vi "FXP_AFMss_LinearDistEst_singleAxis.vi"() -> ()   [LabVIEW 2017]
uses:
  typeDefs/FXPControlParams_distEst.ctl
  fpga_fp_interface_lib/fpga_interface_types/boolean_indicators.ctl
  <vilib>/Platform/TimedLoop/XDataNode/timing_clust.ctl
  <vilib>/Platform/TimedLoop/XDataNode/nitl_modes.ctl
  <vilib>/Platform/TimedLoop/XDataNode/wakeup.ctl
  <vilib>/rvi/Emulation/niFpgaSctlEmulationGetInTimedLoop.vi
  <vilib>/rvi/Emulation/niFpgaProcessEmulError.vi
  <vilib>/rvi/Emulation/niFpgaGetClockAttributes.vi
  <vilib>/rvi/Emulation/niFpgaEmulationReportErrorSimple.vi
  <vilib>/rvi/eio/common/nirviEmuTemplateMethod_errors.vi
  <vilib>/rvi/Emulation/niFpgaCriticalErrorInLSC.vi
  <vilib>/rvi/Memory/Memory_Emulation/nirvimemoryFastEmulation.vi
  <vilib>/rvi/Memory/Memory_Emulation/nirvimemoryEmulation.vi
  <vilib>/rvi/Emulation/niFpgaEmulationIsFPGAContextNoSignature.vi
  <vilib>/rvi/DataTransferAndStorage/Container/Common/niFpgaContainerGetUniqueNameForEmu.vi
  <vilib>/rvi/errors/nirviReportUnexpectedCaseInternalError (U32).vi
  <vilib>/rvi/interface/RandomDataEmulation/niFpgaRandomDataHandleErrors.vi
  <vilib>/eio/EIONode/EIONode.xnode
  <vilib>/Platform/TimedLoop/XDataNode/XDataNode.xnode
  <vilib>/rvi/DataTransferAndStorage/Container/XNode/niFpgaContainer.xnode
  <vilib>/rvi/interface/RandomDataEmulation/nirviRandomDataFpgaReadWriteTemplate.vi
  <vilib>/rvi/FXPMathLib/FxpSub/XNode/nifxpmath_Sub.xnode
  <vilib>/Platform/TimedLoop/XDataNode/XDNodeRunTimeDep.lvlib
  <vilib>/rvi/FXPMathLib/sim/FxpSim.dll
panel:
  out "u_k (saturated)":fxp<+/-,32,5>
  out "del u(k)":fxp<+/-,64,15>
  in  "N_sat":u8
  in  "N_hyst":u8
  in  "Num":sgl[](array[numeric])=[-0.00254, 0.000408, 0.00295, 0.0, 0.0, 0.0, 0.0, 0.0, 0.0]
  in  "Den":sgl[](array[numeric])=[0.982758, -1.98194, 1.0, 0.0, 0.0, 0.0, 0.0, 0.0, 0.0]
  in  "TF Order":i32=2
  out "SS FIFO TimeOut?":bool
  out "u_k":fxp<+/-,32,5>
  out "boolean indicators":T1
  in  "ControlParamsMpc":T2={"umax"=3.0, "Ns_obs/cntrl"=0, "ref_f_VEC"=[0.0, 0.0], "du_max"=0.0, "Nbar"=0.0}
  out "x(0)":fxp<+/-,16,5>
  out "Stopped":bool
  in  "Settle Ticks":i16=1000
  in  "iters":i32=1
  in  "ymax":fxp<+/-,32,16>=4.0
  in  "TsTicks":i16
  out "Loop Ticks (benchmark)":i16
  out "NS_O/C":u8=2
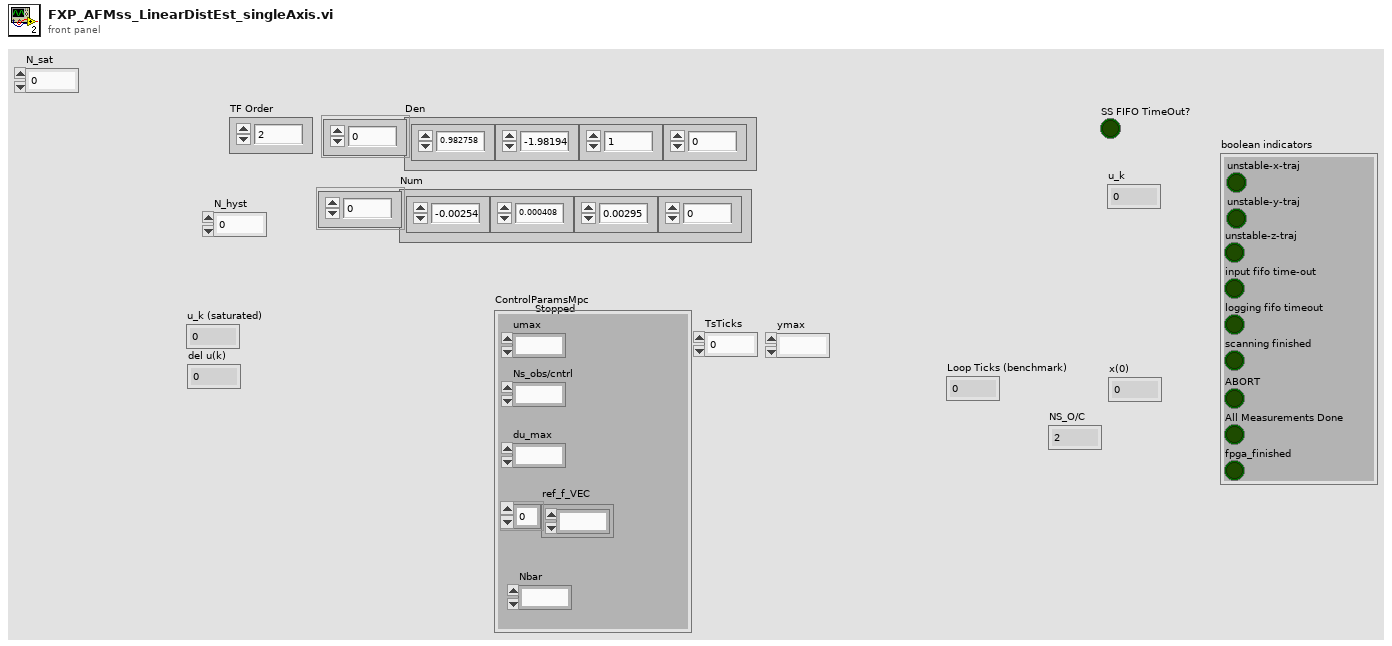
[diagram p1: front panel]
types:
  T1 = typedef "boolean_indicators.ctl" = cluster{"unstable-z-traj":bool, "input fifo time-out":bool, "logging fifo timeout":bool, "scanning finished":bool, "unstable-x-traj":bool, "unstable-y-traj":bool, "ABORT":bool, "All Measurements Done":bool, "fpga_finished":bool}
  T2 = typedef "FXPControlParams_distEst.ctl" = cluster{"umax":fxp<+/-,18,5>, "Ns_obs/cntrl":u8, "ref_f_VEC":fxp<+/-,32,5>[], "du_max":fxp<+/-,18,5>, "Nbar":fxp<+/-,32,5>}
  T3 = typedef "XDNodeRunTimeDep.lvlib/timing_clust.ctl" = cluster{"Expected End [f-1]":u64, "Actual End [f-1]":u64, "Finished Late? [f-1]":bool, "Expected End [i-1]":u64, "Actual End [i-1]":u64, "Finished Late? [i-1]":bool, "Expected Start [i]":u64, "Actual Start [i]":u64, "Expected Start [f]":u64, "Actual Start [f]":u64, "Source Name":string, "Structure Name":string, "Period":i64, "Deadline":i64, "Offset":i64, "Start":i64, "Priority":i32, "Timeout":i32, "Mode":T4, "Wakeup Reason":T5, "Error":errorcluster, "Source Type":string, "Secondary Source Type":string, "Global End Time":u64, "Global Start Time":u64, "Frame Duration":u64, "Iteration Duration":u64, "Assigned CPU":i32, "I/O Scan Engine Mode":u32}
  T4 = typedef "XDNodeRunTimeDep.lvlib/nitl_modes.ctl" = enum32{"No Change", "Process missed periods, maintain original phase", "Discard missed periods, maintain original phase", "Process missed periods, ignore original phase", "Discard missed periods, ignore original phase"}
  T5 = typedef "XDNodeRunTimeDep.lvlib/wakeup.ctl" = enum32{"Normal", "Aborted", "Asynchronous wakeup", "Timing source error", "Timed loop error", "Timeout"}
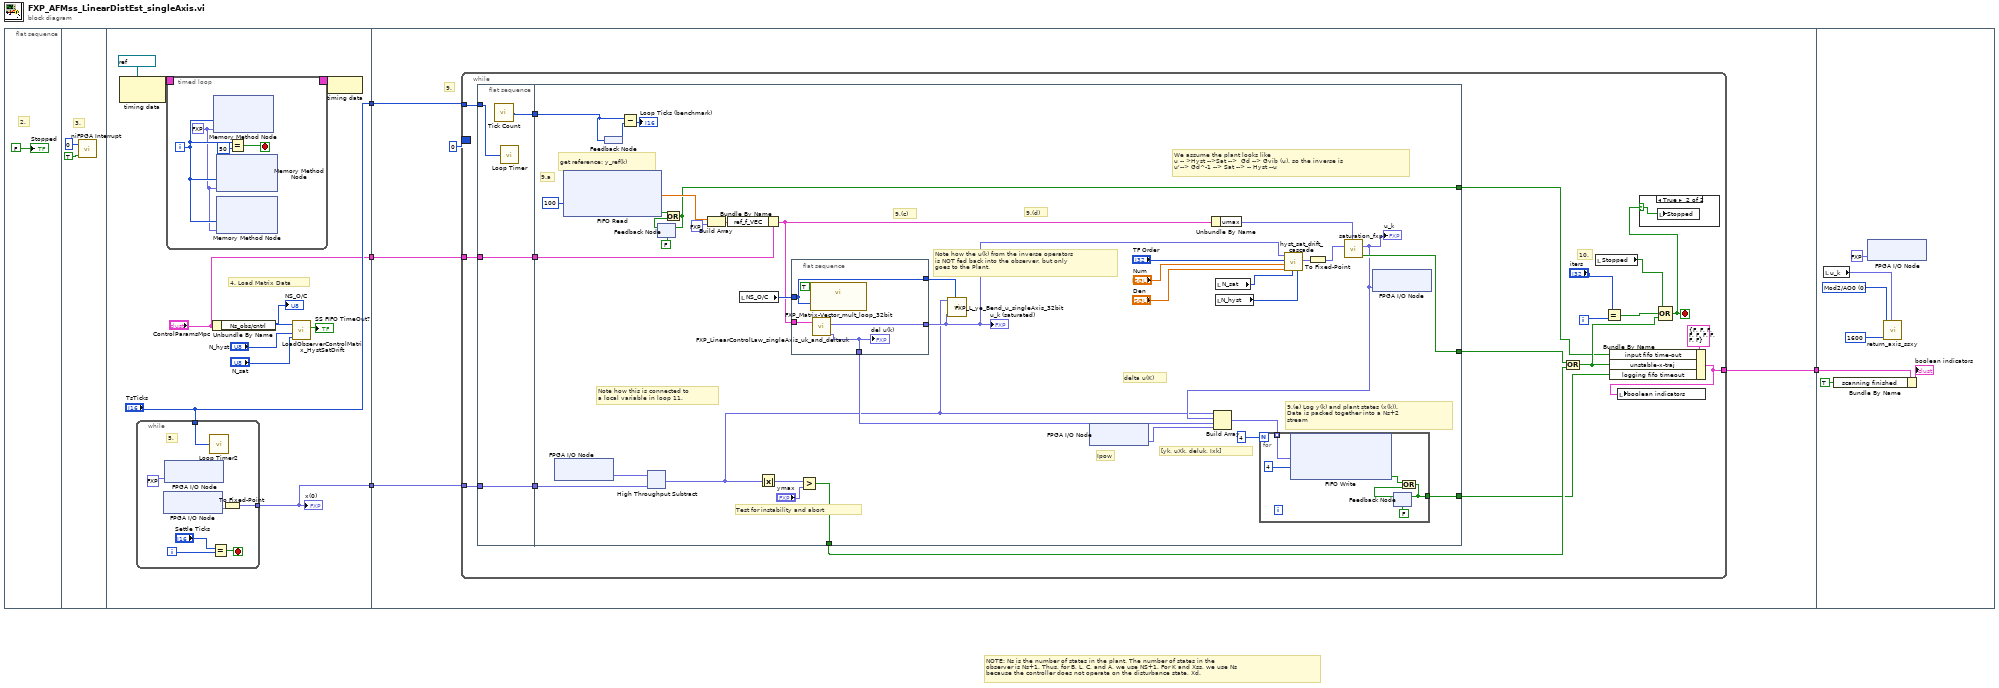
[diagram p0: block diagram]
diagram:
  # "NOTE: Ns is the number of states in the plant. The number of states in the \nobserver is Ns+1. Thus, for B, L, C, and A, we use NS+1. For K and Xss, we use Ns\nbecause the controller does not operate on the disturbance state, Xd."
  n1 = flat-sequence {
    tunnel: ["TsTicks"] -> w4
    tunnel: [w17] -> w3
    tunnel: ["ControlParamsMpc"] -> w2
    tunnel: w4 -> [w39]
    tunnel: w3 -> [w38]
    tunnel: w2 -> [w37]
    tunnel: [w36] -> w1
    tunnel: w1 -> [w116]
    frame #0 {
      # "2."
      "Stopped" <- FALSE ("Stopped")
    }
    frame #1 {
      # "3."
      n2 = call <vilib>:"niFPGA Interrupt.vi"("Wait Until Cleared (F)"=TRUE, "IRQ Number (0)"=u8 0) -> ()  [unwired: 1 in]
    }
    frame #2 {
      # "6."
      # "4. Load Matrix Data"
      n3 = node-c288(refnum<k21> "80MHz" ("Source Name")) -> (w15:T3)
      n4 = while {
        tunnel: [w32] -> w17
        tunnel: "TsTicks" -> [w34]
        i -> [w28]
        stop <- w30 stop-if-true
        # "5."
        n5 = xnode "FPGA I/O Node"() -> ("Mod2/AI0"=w33:fxp<+/-,24,5>)  [unwired: 1 in, 1 out]
        n6 = xnode "FPGA I/O Node"("Mod1/AO0"=fxp<+,1,1> 0.0) -> ()  [unwired: 1 in, 1 out]
        n7 = call "Loop Timer2"("Count(Ticks)"=w34) -> ()  [unwired: 1 out]
        n8 = Equal?(x="Settle Ticks", y=w28) -> (x = y?=w30:bool)
        n9 = To Fixed-Point(number=w33) -> (fixed-point=w32:fxp<+/-,16,5>)  [unwired: 1 in]
      }
      "x(0)" <- w17
      n10 = timed-loop {
        timing: w15 -> [_]
        timing-out: [_] -> w14
        i -> [w19]
        stop <- w21 stop-if-true
        w18 = fxp<+/-,32,5> 0.0 ("Data")
        n11 = xnode ("Memory Method Node")("Address"=w19, "Data"=w18) -> ()  [unwired: 1 in, 1 out]
        n12 = xnode ("Memory Method Node")("Address"=w19, "Data"=w18) -> ()  [unwired: 1 in, 1 out]
        n13 = xnode ("Memory Method Node")("Address"=w19, "Data"=w18) -> ()  [unwired: 1 in, 1 out]
        n14 = Equal?(x=w19, y=50) -> (x = y?=w21:bool)
      }
      n15 = Unbundle By Name("ControlParamsMpc") -> ("Ns_obs/cntrl"=w10:u8)
      "NS_O/C" <- w10
      n16 = call "LoadObserverControlMatrix_HystSatDrift.vi"("Nsat"="N_sat", "Nhyst"="N_hyst", "NS_obs/cntrl"=w10) -> ("SS FIFO TimeOut?"=→"SS FIFO TimeOut?":bool)  [unwired: 8 in]
      n17 = node-c288(w14) -> ()
    }
    frame #3 {
      # "9."
      n18 = while {
        border: i16 0 -> [_]
        tunnel: w37 -> [w55]
        tunnel: w38 -> [w53]
        tunnel: w39 -> [w49]
        tunnel: [w45] -> w36
        i -> [w56]
        stop <- w42 stop-if-true
        # "10."
        n19 = flat-sequence {
          tunnel: w53 -> [w61]
          tunnel: w55 -> [w62]
          tunnel: [w62] -> w52
          tunnel: [w61] -> w51
          tunnel: [w60] -> w50
          tunnel: w49 -> [w59]
          tunnel: [w98] -> w46
          tunnel: w50 -> [w97]
          tunnel: w51 -> [w92]
          tunnel: w52 -> [w77]
          tunnel: [w99] -> w41
          tunnel: [w81] -> w47
          tunnel: [w82] -> w40
          frame #0 {
            n20 = call "Tick Count"() -> ("Tick Count(Ticks)"=w60:u32)
            n21 = call "Loop Timer"("Count(Ticks)"=w59) -> ()  [unwired: 1 out]
          }
          frame #1 {
            # "[yk, uXk, deluk, Ixk]"
            # "Ipow"
            # "We assume the plant looks like\nu -- >Hyst -->Sat -->  Gd --> Gvib (u), so the inverse is\nu'--> Gd^-1 --> Sat --> -- Hyst --u"
            # "get reference: y_ref(k)"
            # "Note how the u(k) from the inverse operators\nis NOT fed back into the observer, but only \ngoes to the Plant."
            # "delta u(K)"
            # "Note how this is connected to\na local variable in loop 11."
            # "9.a"
            # "9.(c)"
            # "9.(d)"
            # "9.(e) Log y(k) and plant states (x(k)). \nData is packed together into a Ns+2 \nstream"
            # "Test for instability and abort"
            n22 = xnode "FPGA I/O Node"() -> ("Mod2/AI0"=w75:fxp<+/-,24,5>)  [unwired: 1 in, 1 out]
            n23 = xnode ("FIFO Read")("Timeout"=i16 100) -> ("Element"=w83:sgl, "Timed Out?"=w86:bool)  [unwired: 1 in, 1 out]
            n24 = feedback #1() -> (w93:u32)
            n25 = feedback-in #1(w97) -> ()
            n26 = Subtract(x=w97, y=w93) -> (x-y=→"Loop Ticks (benchmark)":u32)
            n27 = xnode ("High Throughput Subtract")("x"=w75, "y"=w92) -> ("x-y"=w70:fxp<+/-,18,5>)
            n28 = feedback #2(FALSE) -> (w87:bool)
            n29 = Or(x=w86, y=w87) -> (x .or. y?=w82:bool)
            n30 = feedback-in #2(w82) -> ()
            n31 = Build Array(w83, fxp<+,1,1> 0.0) -> (w85:sgl[])
            n32 = Bundle By Name(cluster=w77, "ref_f_VEC"=w85) -> (w69:T2)
            n33 = local read "NS_O/C"() -> (w78:u8)
            n34 = Absolute Value(x=w70) -> (abs(x)=w96:fxp<+,18,5>)
            n35 = flat-sequence {
              tunnel: w78 -> [w102]
              tunnel: w69 -> [w104]
              tunnel: [w103] -> w76
              tunnel: [w102] -> w72
              tunnel: [w101] -> w71
              frame #0 {
                n36 = call "FXP_Matrix-Vector_mult_loop_32bit.vi"("Ns_1"=w102, "inputValid"=TRUE) -> ()  [unwired: 9 in, 1 out]
                n37 = call "FXP_LinearControlLaw_singleAxis_uk_and_deltauk.vi"("ControlParams_distEst"=w104) -> ("del u_x"=w103:fxp<+/-,64,15>, "u_k (un saturated)"=w101:fxp<+/-,32,5>)  [unwired: 9 in]
                "del u(k)" <- w103
              }
            }
            n38 = Greater?(x=w96, y="ymax") -> (0:w98:bool)
            n39 = call "FXP_L_ye_Bend_u_singleAxis_32bit.vi"("NS"=w72, "U(k): ux"=w71, "Y(k): x"=w70) -> ()  [unwired: 7 in, 2 out]
            n40 = xnode "FPGA I/O Node"() -> ("Mod2/AI2"=w73:fxp<+/-,24,5>)  [unwired: 1 in, 1 out]
            n41 = Unbundle By Name(w69) -> ("umax"=w79:fxp<+/-,18,5>)
            n42 = local read "N_hyst"() -> (w66:u8)
            n43 = local read "N_sat"() -> (w67:u8)
            n44 = call "hyst_sat_drift_cascade.vi"("N_hyst"=w66, "N_sat"=w67, "Den"="Den", "Num"="Num", "TF Order"="TF Order", "u_k (un saturated)"=w71) -> ("Hinv(uk)"=w63:fxp<+/-,32,10>)  [unwired: 5 in]
            n45 = To Fixed-Point(number=w63) -> (fixed-point=w80:fxp<+/-,32,5>)  [unwired: 1 in]
            n46 = call "saturation_fxp.vi"("uMax"=w79, "signal_in"=w80) -> ("has_saturated"=w81:bool, "signal_out (saturated)"=w74:fxp<+/-,32,6>)  [unwired: 8 in]
            "u_k" <- w74
            n47 = Build Array(w70, w74, w76, w73) -> (w91:fxp<+/-,64,15>[])
            n48 = for {
              N: i16 4 -> [_]
              tunnel: w91 -> [w109] mode=indexing
              tunnel: [w105] -> w99
              n49 = xnode ("FIFO Write")("Element"=w109, "Timeout"=i16 4) -> ("Timed Out?"=w108:bool)  [unwired: 1 in, 1 out]
              n50 = feedback #3(FALSE) -> (w107:bool)
              n51 = Or(x=w108, y=w107) -> (x .or. y?=w105:bool)
              n52 = feedback-in #3(w105) -> ()
            }
            n53 = xnode "FPGA I/O Node"("Mod1/AO0"=w74) -> ()  [unwired: 1 in, 1 out]
            "u_k (saturated)" <- w71
          }
        }
        n54 = Or(x=w47, y=w46) -> (x .or. y?=w43:bool)
        n55 = local read "Stopped"() -> (w44:bool)
        n56 = Equal?(x="iters", y=w56) -> (x = y?=w54:bool)
        n57 = Bundle By Name(cluster=T1 {"unstable-z-traj"=FALSE, "input fifo time-out"=FALSE, "logging fifo timeout"=FALSE, "scanning finished"=FALSE, "unstable-x-traj"=FALSE, "unstable-y-traj"=FALSE, "ABORT"=FALSE, "All Measurements Done"=FALSE, "fpga_finished"=FALSE} ("boolean  indicators"), "input fifo time-out"=w40, "unstable-x-traj"=w43, "logging fifo timeout"=w41) -> (w45:T1)
        n58 = local write "boolean indicators"(w45) -> ()
        n59 = Compound Arithmetic op=OR(w44, w54, w43) -> (w42:bool)
        n60 = case shown="True" w42 {
          selector: w42 -> [_ w58]
          frame False {
          }
          frame True {
            n61 = local write "Stopped"(w58) -> ()
          }
        }
      }
    }
    frame #4 {
      w112 = i16 0 items=["Mod2/AO0", "Mod2/AO1", "Mod2/AO2", "Mod2/AO3", ""] ("DAC-select")
      n62 = local read "u_k"() -> (w111:fxp<+/-,32,5>)
      n63 = Bundle By Name(cluster=w116, "scanning finished"=TRUE) -> (→"boolean indicators":T1)
      n64 = xnode "FPGA I/O Node"("Mod1/AO1"=fxp<+/-,20,5> 0.0 ("Mod1/AO0")) -> ()  [unwired: 1 in, 1 out]
      n65 = call "return_axis_ssxy.vi"("u(0)"=w111, "TsTicks"=u32 1600, "DAC-select"=w112) -> ()  [unwired: 9 in]
    }
  }
